vi "blueScreenTestPixelfly.vi"() -> ()   [LabVIEW 2009, in "run.lvlib"]
uses:
  run.lvlib
  Channels/Camera/PixelflySA/PixelflySA.lvclass
  Tools/Filing/FileSystem/FileSystem.lvclass
  Tools/CameraSettings/CamaraSettings.lvclass
  Tools/Filing/FileNeologist/FileNeologist.lvclass
panel:
  out "stopped?":bool
  in  "stop":bool
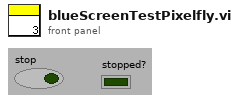
[diagram p1: front panel]
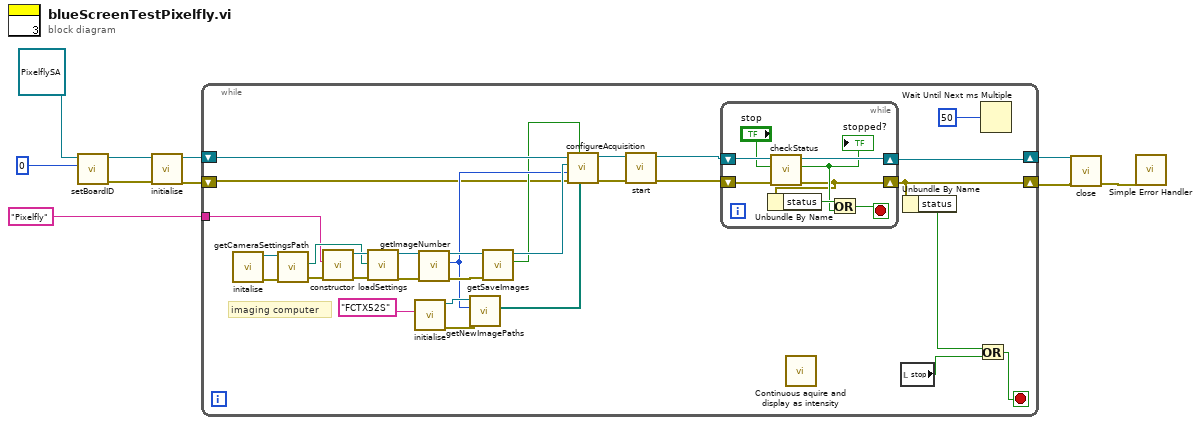
[diagram p0: block diagram]
diagram:
  n1 = call "setBoardID.vi"("boardID"=0, "Pixelfly in"=refnum<class "PixelflySA.lvclass"> refnum) -> ("error out"=w4:errorcluster, "Pixelfly out"=w5:refnum<class "PixelflySA.lvclass">)  [unwired: 8 in]
  n2 = call "initialise.vi"("error in (no error)"=w4, "Pixelfly in"=w5) -> ("error out"=w6:errorcluster, "Pixelfly out"=w7:refnum<class "PixelflySA.lvclass">)  [unwired: 8 in]
  n3 = while {
    tunnel: "Pixelfly" -> [w27]
    shift-right: [w22] -> w2
    shift-left: w6 -> [w15]
    shift-right: [w21] -> w3
    shift-left: w7 -> [w20]
    stop <- w26 stop-if-true
    # "imaging computer"
    n4 = call "initalise.vi"() -> ("error out"=w39:errorcluster, "FileSystem out"=w40:refnum<class "FileSystem.lvclass">)  [unwired: 10 in]
    n5 = call-dynamic "getCameraSettingsPath.vi"("error in (no error)"=w39, "FileSystem.lvclass in"=w40) -> ("error out"=w37:errorcluster, "CameraSettingsPath"=w36:path)  [unwired: 7 in, 1 out]
    n6 = call "constructor.vi"("error in (no error)"=w37, "camera settings"=w27) -> ("error out"=w35:errorcluster, "CamaraSettings out"=w38:refnum<class "CamaraSettings.lvclass">)  [unwired: 8 in]
    n7 = call-dynamic "loadSettings.vi"("error in (no error)"=w35, "Path"=w36, "CamaraSettings in"=w38) -> ("error out"=w33:errorcluster, "CamaraSettings out"=w34:refnum<class "CamaraSettings.lvclass">)  [unwired: 7 in]
    n8 = call "initialise.vi"("computer name"="FCTX52S") -> ("error out"=w29:errorcluster, "FileNeologist out"=w30:refnum<class "FileNeologist.lvclass">)  [unwired: 9 in]
    n9 = call-dynamic "getImageNumber.vi"("error in (no error)"=w33, "CamaraSettings in"=w34) -> ("error out"=w31:errorcluster, "image number"=w18:i32, "CamaraSettings out"=w32:refnum<class "CamaraSettings.lvclass">)  [unwired: 7 in]
    n10 = call "getNewImagePaths.vi"("error in (no error)"=w29, "numberOfImages"=w18, "FileNeologist in"=w30) -> ("Paths"=w16:path[])  [unwired: 6 in, 2 out]
    n11 = call "getSaveImages.vi"("error in (no error)"=w31, "CamaraSettings in"=w32) -> ("saveImages"=w17:bool, "CamaraSettings out"=w19:refnum<class "CamaraSettings.lvclass">)  [unwired: 7 in, 1 out]
    n12 = call "configureAcquisition.vi"("imagePaths"=w16, "saveImages?"=w17, "error in (no error)"=w15, "number of Images"=w18, "CameraSettings"=w19, "Pixelfly in"=w20) -> ("error out"=w14:errorcluster, "Pixelfly out"=w13:refnum<class "PixelflySA.lvclass">)  [unwired: 4 in]
    n13 = call "start.vi"("error in (no error)"=w14, "Pixelfly in"=w13) -> ("error out"=w11:errorcluster, "Pixelfly out"=w12:refnum<class "PixelflySA.lvclass">)  [unwired: 8 in]
    n14 = while {
      shift-right: [w41] -> w22
      shift-left: w11 -> [w45]
      shift-right: [w43] -> w21
      shift-left: w12 -> [w46]
      stop <- w47 stop-if-true
      n15 = call "checkStatus.vi"("error in (no error)"=w45, "stop"="stop", "Pixelfly in"=w46) -> ("error out"=w41:errorcluster, "stopped?"=w42:bool, "Pixelfly out"=w43:refnum<class "PixelflySA.lvclass">)  [unwired: 6 in]
      "stopped?" <- w42
      n16 = Unbundle By Name(w41) -> ("status"=w48:bool)
      n17 = Or(x=w48, y=w42) -> (x .or. y?=w47:bool)
    }
    n18 = call <instrlib>:"Continuous aquire and display as intensity.vi"() -> ()  [unwired: 1 in]
    n19 = local read "stop"() -> (w24:bool)
    n20 = Unbundle By Name(w22) -> ("status"=w25:bool)
    n21 = Or(x=w25, y=w24) -> (x .or. y?=w26:bool)
    n22 = Wait Until Next ms Multiple(millisecond multiple=50) -> ()  [unwired: 1 out]
  }
  n23 = call "close.vi"("error in (no error)"=w2, "Pixelfly in"=w3) -> ("error out"=w1:errorcluster)  [unwired: 9 in]
  n24 = call <vilib>:"Simple Error Handler.vi"("error in (no error)"=w1) -> ()  [unwired: 4 in, 5 out]
